vi "Read-Test Instrument.vi"(4 "Data Array In":dbl[](array[numeric]), 5 "Action":T1=enum."Read", 7 "Instrument Prop":T2={"Public"={"Column Name"=[], "Trace Color"=[]}, "Private"={"Path"=path "", "VI Refnum"=refnum, "Name"="", "# of Values"=0, "Scale Factors"=[], "Display"=[], "Offset"=[1.0]}} {"Private"."Offset" format="%^_3e"; "Private"."Scale Factors" format="%^_3e"}) -> (0 "Stop":bool, 2 "Data Array Out":dbl[](array[numeric]), 3 "Instrument Prop 2":T2={"Public"={"Column Name"=[], "Trace Color"=[]}, "Private"={"Path"=path "", "VI Refnum"=refnum, "Name"="", "# of Values"=0, "Scale Factors"=[], "Display"=[], "Offset"=[1.0]}} {"Private"."Offset" format="%^_3e"; "Private"."Scale Factors" format="%^_3e"})   [LabVIEW 2020]
uses:
  Sub Controls/Instrument Properties.ctl
  Sub Controls/Public.ctl
  Sub Controls/Private.ctl
  Sub Controls/Instrument Ref.ctl
  Sub Controls/SystemCheckBox-resize.ctl
  Sub Controls/Instrument Actions.ctl
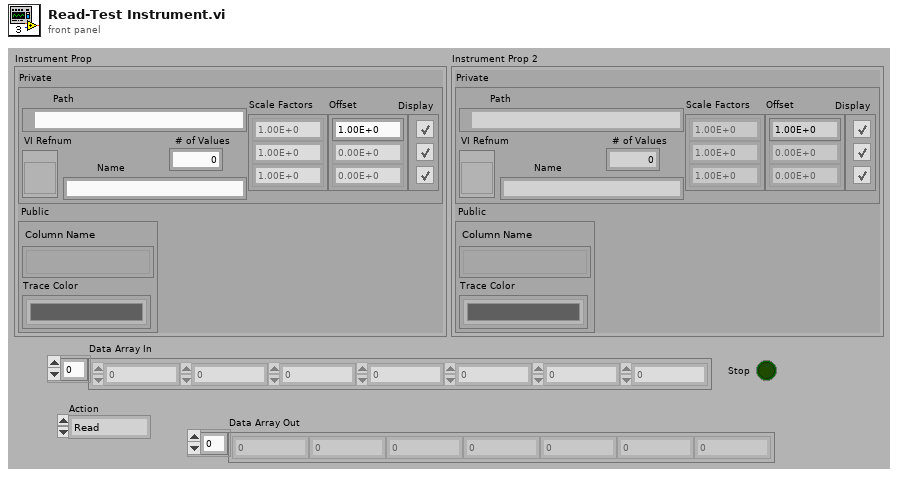
[diagram p1: front panel]
types:
  T1 = typedef "Instrument Actions.ctl" = enum16{"Scan", "Identify", "New", "Configure", "Initialize", "Test", "Read", "Close"}
  T2 = typedef "Instrument Properties.ctl" = cluster{"Public":T3, "Private":T4}
  T3 = typedef "Public.ctl" = cluster{"Column Name":string[], "Trace Color":u32[]}
  T4 = typedef "Private.ctl" = cluster{"Path":path, "VI Refnum":T5, "Name":string, "# of Values":i32, "Scale Factors":dbl[], "Display":T6[], "Offset":dbl[]}
  T5 = typedef "Instrument Ref.ctl" = refnum<vi>
  T6 = typedef "SystemCheckBox-resize.ctl" = bool
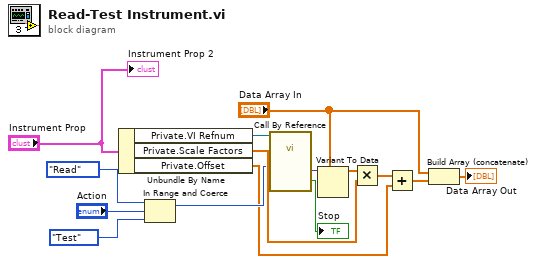
[diagram p0: block diagram]
diagram:
  n1 = Unbundle By Name("Instrument Prop") -> ("Private.VI Refnum"=w15:T5, "Private.Scale Factors"=w7:dbl[], "Private.Offset"=w1:dbl[])
  n2 = In Range and Coerce(upper limit=Instrument_Actions."Read", x="Action", lower limit=Instrument_Actions."Test") -> (coerced(x)=w5:T1)  [unwired: 1 out]
  n3 = call-by-ref "?"(reference=w15, "Action"=w5) -> ("Output"=w13:variant, "Stop"=→"Stop":bool)  [unwired: 6 in, 2 out]
  n4 = Variant To Data(type="Data Array In", Variant=w13) -> (data=w10:dbl[])  [unwired: 1 in, 1 out]
  n5 = Multiply(x=w10, y=w7) -> (x*y=w8:dbl[])
  n6 = Add(x=w8, y=w1) -> (x+y=w2:dbl[])
  n7 = Build Array (concatenate)("Data Array In", w2) -> (→"Data Array Out":dbl[])
  "Instrument Prop 2" <- "Instrument Prop"
